vi "SaveDataLog.vi"(2 "entrée d'erreur":errorcluster, 3 "DataLoggingCluster":T1 {"Add. Param. No 2" format="%#_6f"; "Add. Param. No 1" format="%#_6f"; "Wedge Insertion (mm)" format="%#_6f"; "Pulse Duration (fs)" format="%#_6f"; "Parabola Position (um)" format="%#_6f"; "Pulse Energy (mJ)" format="%#_6f"; "Chirp (fs^2)" format="%#_6f"}, 4 "chemin du fichier (utiliser une boîte de dialogue)":path) -> (0 "sortie d'erreur":errorcluster)   [LabVIEW 2015, in "ShhgDataLogging.lvlib"]
uses:
  ShhgDataLogging.lvlib
  DataLoggingCluster.ctl
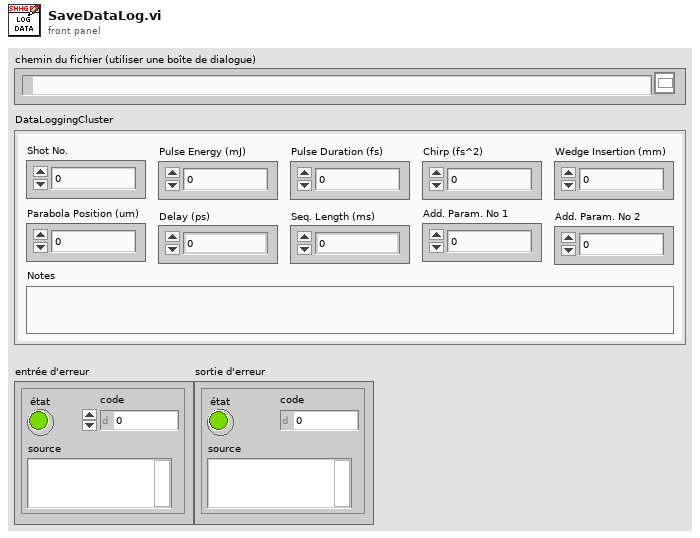
[diagram p1: front panel]
types:
  T1 = typedef "ShhgDataLogging.lvlib/DataLoggingCluster.ctl" = cluster{"Shot No. ":u32, "Pulse Energy (mJ)":dbl, "Pulse Duration (fs)":dbl, "Chirp (fs^2)":dbl, "Wedge Insertion (mm)":dbl, "Parabola Position (um)":dbl, "Delay (ps)":dbl, "Seq. Length (ms)":dbl, "Add. Param. No 1":dbl, "Add. Param. No 2":dbl, "Notes":string}
  T2 = enum16{"open", "replace", "create", "open or create", "replace or create", "replace or create with confirmation"}
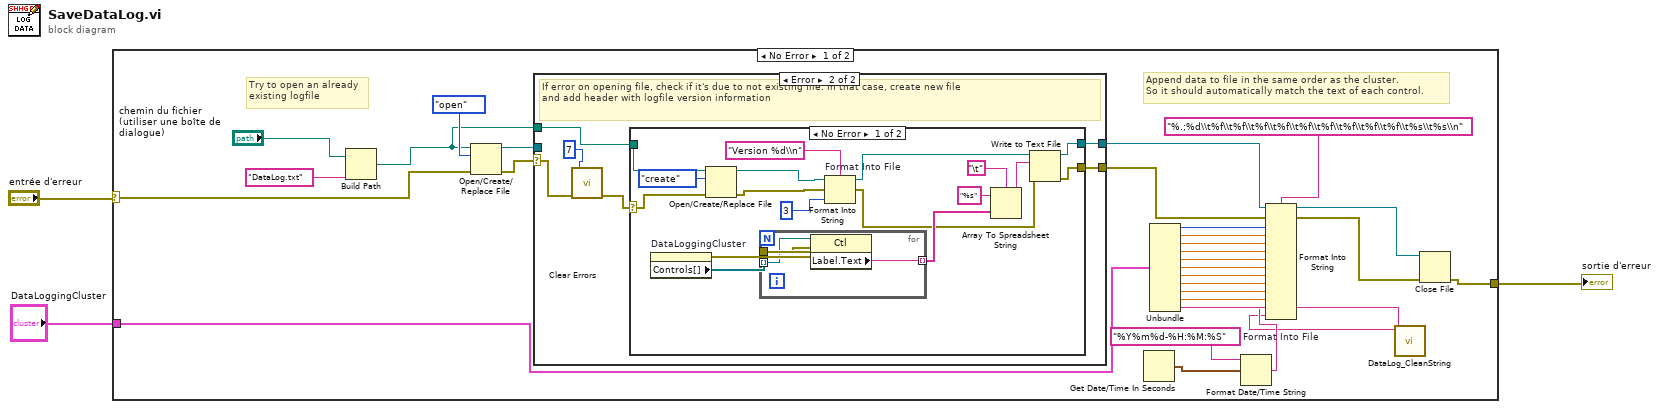
[diagram p0: block diagram]
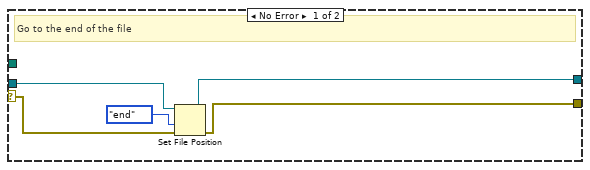
[diagram p2: hidden frame]
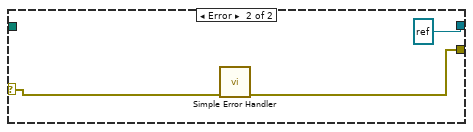
[diagram p3: hidden frame]
diagram:
  n1 = case shown="No Error" "entrée d'erreur" {
    selector: "entrée d'erreur" -> [w21 w67]
    tunnel: [w30 w67] -> w3
    tunnel: "DataLoggingCluster" -> [w19 _]
    frame No Error {
      # "Append data to file in the same order as the cluster.\nSo it should automatically match the text of each control."
      # "Try to open an already\nexisting logfile"
      n2 = Build Path(base path="chemin du fichier (utiliser une boîte de dialogue)", name or relative path="DataLog.txt") -> (appended path=w20:path)
      n3 = Open/Create/Replace File(file path (use dialog)=w20, error in=w21, operation (0:open)=T2."open" ("opération (0 : open)")) -> (refnum out=w24:refnum<file>, error out=w25:errorcluster)  [unwired: 3 in, 1 out]
      n4 = case shown="Error" w25 {
        selector: w25 -> [w37 w43]
        tunnel: w24 -> [w35 _]
        tunnel: [w34 w40] -> w23
        tunnel: [w33 w38] -> w22
        tunnel: w20 -> [_ w39]
        frame No Error {
          # "Go to the end of the file"
          n5 = Set File Position(refnum=w35, from (0:start)=enum16{"start", "end", "current"}."end" ("à partir de (0 : start)"), error in=w37) -> (refnum out=w33:refnum<file>, error out=w34:errorcluster)  [unwired: 1 in]
        }
        frame Error {
          # "If error on opening file, check if it's due to not existing file. In that case, create new file \nand add header with logfile version information"
          n6 = call <vilib>:"Clear Errors.vi"("error in (no error)"=w43, "specific error code to clear (0: all)"=7) -> ("error out"=w41:errorcluster)  [unwired: 4 in, 1 out]
          n7 = case shown="No Error" w41 {
            selector: w41 -> [w60 w65]
            tunnel: [w46 w64] -> w40
            tunnel: w39 -> [w59 _]
            tunnel: [w45 refnum<file> refnum ("refnum out")] -> w38
            frame No Error {
              n8 = property on="DataLoggingCluster" class="Clust (strict)"() -> (error out=w53:errorcluster, "Controls[]"=w52:refnum<vi>[])  [unwired: 2 in, 1 out]
              n9 = Open/Create/Replace File(file path (use dialog)=w59, error in=w60, operation (0:open)=T2."create") -> (refnum out=w56:refnum<file>, error out=w55:errorcluster)  [unwired: 3 in, 1 out]
              n10 = for {
                tunnel: w52 -> [w63] mode=indexing
                tunnel: w53 -> [w62]
                tunnel: [w61] -> w51 mode=indexing
                n11 = property class="Ctl"(reference=w63, error in=w62) -> ("Label.Text"=w61:string)  [unwired: 2 out]
              }
              n12 = Format Into String "Format Into File"(format string="Version %d\\n", initial string=w56, error in=w55, u32 3 ("input 1")) -> (resulting string=w48:refnum<file>, error out=w47:errorcluster)
              n13 = Array To Spreadsheet String(delimiter (Tab)="\t", array=w51, 3:"%s" ("format string")) -> (spreadsheet string=w49:string)
              n14 = Write to Text File(file (use dialog)=w48, text=w49, error in=w47) -> (refnum out=w45:refnum<file>, error out=w46:errorcluster)  [unwired: 1 in, 1 out]
            }
            frame Error {
              n15 = call <vilib>:"Simple Error Handler.vi"("error in (no error)"=w65) -> ("error out"=w64:errorcluster)  [unwired: 4 in, 4 out]
            }
          }
        }
      }
      n16 = Get Date/Time In Seconds() -> (seconds since 1Jan1904=w7:timestamp)
      n17 = Unbundle(w19) -> ("Shot No."=w8:u32, "Pulse Energy (mJ)"=w9:dbl, "Pulse Duration (fs)"=w10:dbl, "Chirp (fs^2)"=w11:dbl, "Wedge Insertion (mm)"=w12:dbl, "Parabola Position (um)"=w13:dbl, "Delay (ps)"=w14:dbl, "Seq. Length (ms)"=w15:dbl, "Add. Param. No 1"=w16:dbl, "Add. Param. No 2"=w17:dbl, "Notes"=w18:string)
      n18 = Format Date/Time String(time format string (%c)="%Y%m%d-%H:%M:%S", seconds (now)=w7) -> (date/time string=w5:string)  [unwired: 1 in]
      n19 = call "DataLog_CleanString.vi"("Notes in"=w18) -> ("Notes out"=w4:string)  [unwired: 10 in]
      n20 = Format Into String "Format Into File"(format string="%.;%d\\t%f\\t%f\\t%f\\t%f\\t%f\\t%f\\t%f\\t%f\\t%f\\t%s\\t%s\\n" ("chaîne de format"), initial string=w22, error in=w23, w8, w9, w10, w11, w12, w13, w14, w15, w16, w17, w5, w4) -> (resulting string=w31:refnum<file>, error out=w32:errorcluster)
      n21 = Close File(refnum=w31, error in=w32) -> (error out=w30:errorcluster)  [unwired: 1 out]
    }
    frame Error {
    }
  }
  "sortie d'erreur" <- w3
